vi "Dispose.vi"(8 "error in (no error)":errorcluster, 11 "Actor in":refnum<class "Actor.lvclass">) -> (0 "error out":errorcluster, 3 "Actor out":refnum<class "Actor.lvclass">)   [LabVIEW 2020, in "CameraTesting.lvlib" / "CameraTesting.lvclass"]
uses:
  CameraTesting.lvclass
  CameraTesting.lvclass/CameraTesting.ctl
  <vilib>/ActorFramework/Actor/Actor.lvclass
  C:/Program Files (x86)/National Instruments/LabVIEW 2020/vi.lib/ActorFramework/Actor/Actor.lvclass
  E:/GitHub/Evaluation_Test/Labview/src/CameraTestingApp/CameraTesting/CameraTesting/CameraTesting.lvclass
  E:/GitHub/Evaluation_Test/Labview/src/CameraTestingApp/ICameraTesting/ICameraTesting/ICameraTesting.lvclass
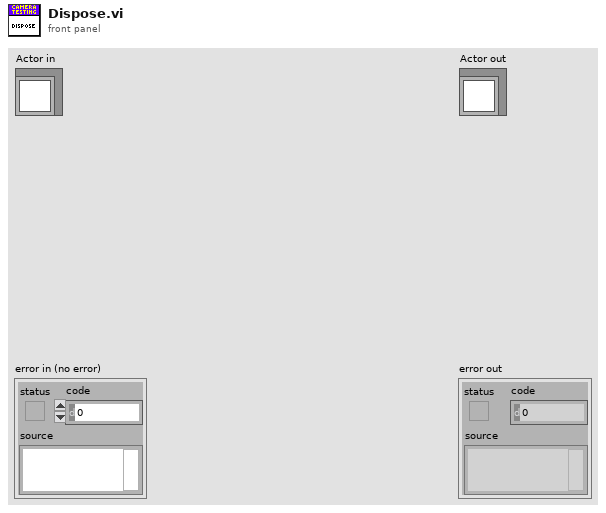
[diagram p1: front panel]
types:
  T1 = typedef "ICameraTesting.lvlib/ICameraTesting.lvclass/FrameRateValReceived.ctl" = refnum<user-event>
  T2 = typedef "ICameraTesting.lvlib/ICameraTesting.lvclass/ImgTypeValReceived.ctl" = refnum<user-event>
  T3 = typedef "ICameraTesting.lvlib/ICameraTesting.lvclass/ResolutionValReceived.ctl" = refnum<user-event>
  T4 = typedef "ICameraTesting.lvlib/ICameraTesting.lvclass/VideoOptCodesUpdated.ctl" = refnum<user-event>
  T5 = typedef "ICameraTesting.lvlib/ICameraTesting.lvclass/StatusUpdated.ctl" = refnum<user-event>
  T6 = typedef "ICameraTesting.lvlib/ICameraTesting.lvclass/VideoBufferUpdate.ctl" = refnum<user-event>
  T7 = typedef "CameraTesting.lvlib/CameraTesting.lvclass/ActorStopped.ctl" = refnum<user-event>
  T8 = typedef "ICamera.lvlib/ICamera.lvclass/StreamDataEvent.ctl" = refnum<user-event>
  T9 = typedef "CameraTesting.lvlib/CameraTesting.lvclass/EvntRegRefnum.ctl" = refnum<event-registration>
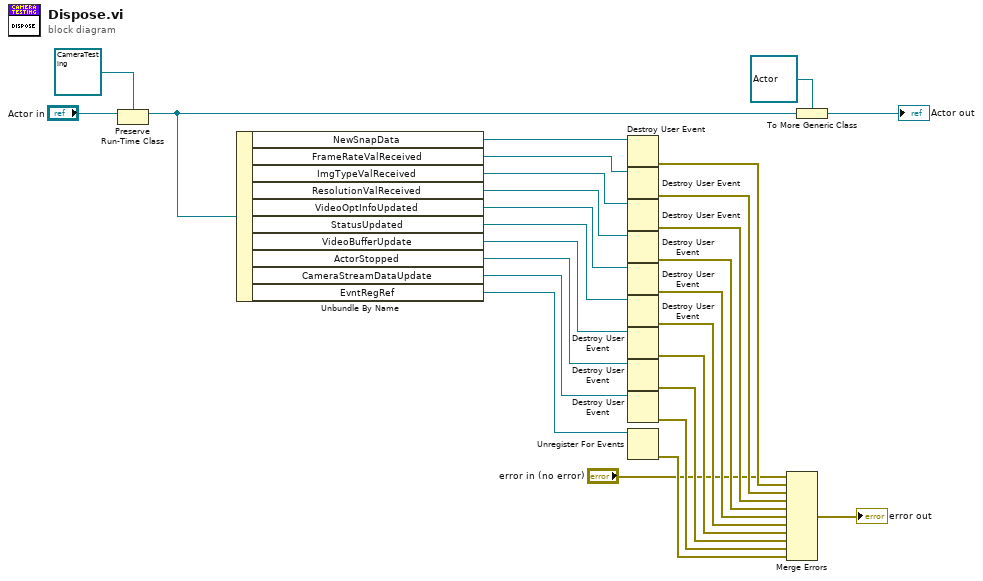
[diagram p0: block diagram]
diagram:
  n1 = Preserve Run-Time Class(object in="Actor in", 2:refnum<class "CameraTesting.lvclass"> refnum ("CameraTesting.lvlib:CameraTesting.lvclass")) -> (object out=w3:refnum<class "CameraTesting.lvclass">)  [unwired: 1 in, 1 out]
  n2 = Unbundle By Name(w3) -> ("NewSnapData"=w27:refnum<user-event>, "FrameRateValReceived"=w26:T1, "ImgTypeValReceived"=w25:T2, "ResolutionValReceived"=w24:T3, "VideoOptInfoUpdated"=w23:T4, "StatusUpdated"=w22:T5, "VideoBufferUpdate"=w21:T6, "ActorStopped"=w20:T7, "CameraStreamDataUpdate"=w19:T8, "EvntRegRef"=w18:T9)
  n3 = Destroy User Event(user event=w27) -> (error out=w17:errorcluster)  [unwired: 1 in]
  n4 = Destroy User Event(user event=w26) -> (error out=w16:errorcluster)  [unwired: 1 in]
  n5 = Destroy User Event(user event=w25) -> (error out=w15:errorcluster)  [unwired: 1 in]
  n6 = Destroy User Event(user event=w24) -> (error out=w14:errorcluster)  [unwired: 1 in]
  n7 = Destroy User Event(user event=w23) -> (error out=w13:errorcluster)  [unwired: 1 in]
  n8 = Destroy User Event(user event=w22) -> (error out=w12:errorcluster)  [unwired: 1 in]
  n9 = Destroy User Event(user event=w21) -> (error out=w11:errorcluster)  [unwired: 1 in]
  n10 = Destroy User Event(user event=w20) -> (error out=w10:errorcluster)  [unwired: 1 in]
  n11 = Destroy User Event(user event=w19) -> (error out=w9:errorcluster)  [unwired: 1 in]
  n12 = Unregister For Events(event registration refnum=w18) -> (error out=w8:errorcluster)  [unwired: 1 in]
  n13 = Merge Errors("error in (no error)", w17, w16, w15, w14, w13, w12, w11, w10, w9, w8) -> (→"error out":errorcluster)
  n14 = To More Generic Class(target class=refnum<class "Actor.lvclass"> refnum ("Actor in"), reference=w3) -> (generic class reference=→"Actor out":refnum<class "Actor.lvclass">)
